vi "Get Wheel Parameter by Name.vi"(8 "error in (no error)":errorcluster, 10 "parameter name":string, 11 "wheel in":refnum<class "NI_Robotics_Wheel.lvclass">) -> (0 "error out":errorcluster, 1 "found?":bool, 2 "parameter value":variant, 3 "wheel out":refnum<class "NI_Robotics_Wheel.lvclass">)   [LabVIEW 2017, in "NI_Robotics_Wheel.lvclass"]
uses:
  <vilib>/robotics/Steering/Wheel/NI_Robotics_Wheel.lvclass
  <vilib>/robotics/Steering/Wheel/NI_Robotics_Wheel.lvclass/NI_Robotics_Wheel.ctl
  <vilib>/robotics/Actuation/Motor Communication/NI_Robotics_Motor Communication.lvclass
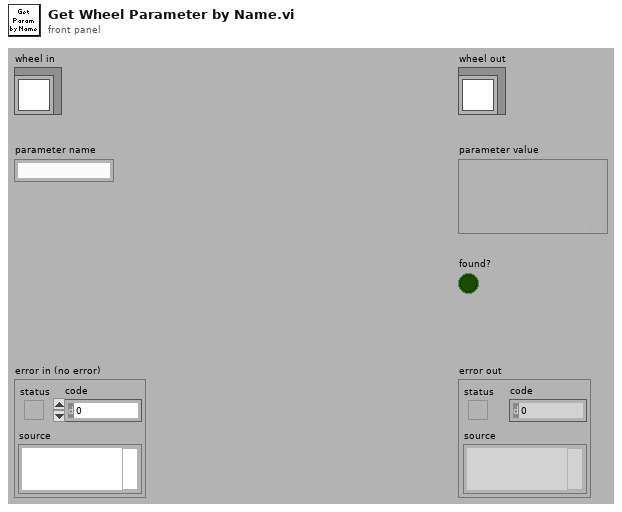
[diagram p1: front panel]
types:
  T1 = typedef "NI_Robotics_Wheel.lvclass/Rotation Direction.ctl" = u16
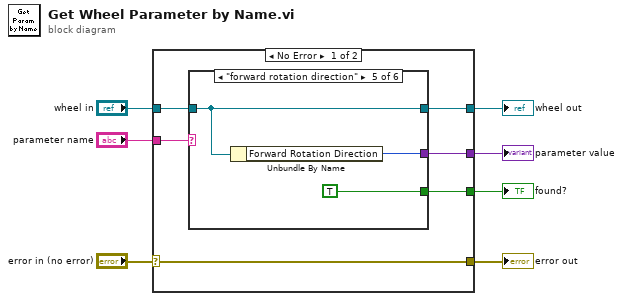
[diagram p0: block diagram]
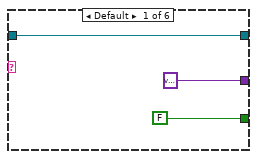
[diagram p2: hidden frame]
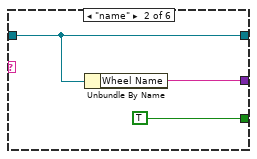
[diagram p3: hidden frame]
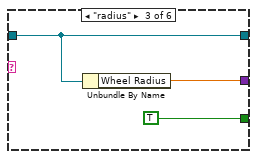
[diagram p4: hidden frame]
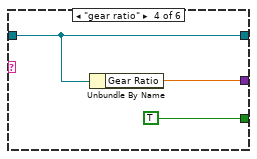
[diagram p5: hidden frame]
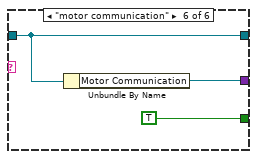
[diagram p6: hidden frame]
diagram:
  n1 = case shown="No Error" "error in (no error)" {
    selector: "error in (no error)" -> [w13 w33]
    tunnel: [w13 w33] -> w6
    tunnel: [w10 w32] -> w4
    tunnel: "wheel in" -> [w11 w32]
    tunnel: "parameter name" -> [w12 _]
    tunnel: [w9 _] -> w2
    tunnel: [w8 _] -> w1
    frame No Error {
      n2 = case shown="\"forward rotation direction\"" w12 {
        tunnel: w11 -> [w16 w19 w22 w25 w28 w31]
        tunnel: [w16 w19 w22 w25 w28 w31] -> w10
        tunnel: [variant ("parameter value") w18 w21 w24 w27 w30] -> w9
        tunnel: [FALSE TRUE TRUE TRUE TRUE TRUE] -> w8
        frame Default {
        }
        frame "name" {
          n3 = Unbundle By Name(w19) -> ("Wheel Name"=w18:string)
        }
        frame "radius" {
          n4 = Unbundle By Name(w22) -> ("Wheel Radius"=w21:dbl)
        }
        frame "gear ratio" {
          n5 = Unbundle By Name(w25) -> ("Gear Ratio"=w24:dbl)
        }
        frame "forward rotation direction" {
          n6 = Unbundle By Name(w28) -> ("Forward Rotation Direction"=w27:T1)
        }
        frame "motor communication" {
          n7 = Unbundle By Name(w31) -> ("Motor Communication"=w30:refnum<class "NI_Robotics_Motor Communication.lvclass">)
        }
      }
    }
    frame Error {
    }
  }
  "error out" <- w6
  "wheel out" <- w4
  "parameter value" <- w2
  "found?" <- w1
